vi "Convert 8SPC to 16SPC.vi"(0 "8xIQ in":T3=[{"I"=0.0, "Q"=0.0, "overflow"=FALSE}, {"I"=0.0, "Q"=0.0, "overflow"=FALSE}, {"I"=0.0, "Q"=0.0, "overflow"=FALSE}, {"I"=0.0, "Q"=0.0, "overflow"=FALSE}, {"I"=0.0, "Q"=0.0, "overflow"=FALSE}, {"I"=0.0, "Q"=0.0, "overflow"=FALSE}, {"I"=0.0, "Q"=0.0, "overflow"=FALSE}, {"I"=0.0, "Q"=0.0, "overflow"=FALSE}], 9 "input valid":bool=TRUE) -> (4 "16xIQ out":T1, 10 "output valid":bool=TRUE)   [LabVIEW 2015, in "DDC_7976R_v1.lvlib"]
uses:
  DDC_7976R_v1.lvlib
  Private/8xIQData.ctl
  <instrlib>/_niInstr/DSP/v1/Shared/Public/IQ Data.ctl
  Private/16xIQData.ctl
  <instrlib>/_niInstr/Basic Elements/v1/FPGA/niInstr Basic Elements v1 FPGA.lvlib
  <instrlib>/_niInstr/DSP/v1/Shared/niInstr DSP v1 Shared.lvlib
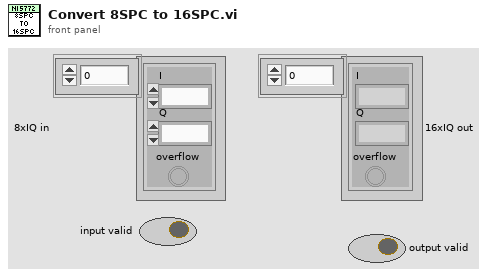
[diagram p1: front panel]
types:
  T1 = typedef "DDC_7976R_v1.lvlib/16xIQData.ctl" = T2[]
  T2 = typedef "niInstr DSP v1 Shared.lvlib/IQ Data.ctl" = cluster{"I":fxp<+/-,18,1>, "Q":fxp<+/-,18,1>, "overflow":bool}
  T3 = typedef "DDC_7976R_v1.lvlib/8xIQData.ctl" = T2[]
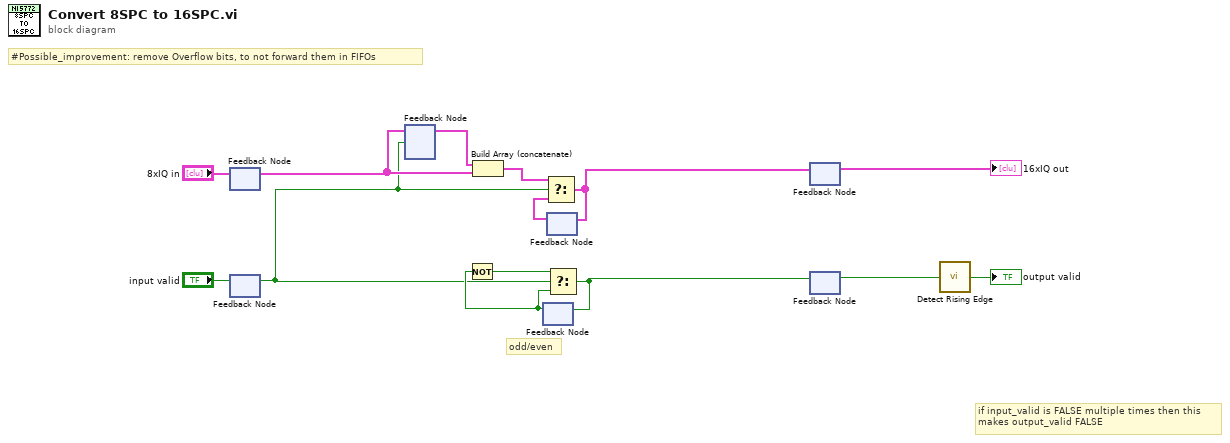
[diagram p0: block diagram]
diagram:
  # "odd/even"
  # "#Possible_improvement: remove Overflow bits, to not forward them in FIFOs"
  # "if input_valid is FALSE multiple times then this\nmakes output_valid FALSE"
  n1 = feedback #1() -> (w11:T3)  [unwired: 1 in]
  n2 = feedback-in #1("8xIQ in") -> ()
  n3 = feedback #2() -> (w1:bool)  [unwired: 1 in]
  n4 = feedback-in #2("input valid") -> ()
  n5 = feedback #3() -> (w8:T3)  [unwired: 1 in]
  n6 = feedback-in #3(w11, w1) -> ()
  n7 = Build Array (concatenate)(w8, w11) -> (w7:T2[])
  n8 = feedback #4() -> (w3:bool)  [unwired: 1 in]
  n9 = Not(x=w3) -> (.not. x?=w4:bool)
  n10 = feedback #5() -> (w6:T2[])  [unwired: 1 in]
  n11 = Select(t=w7, s=w1, f=w6) -> (s? t:f=w5:T2[])
  n12 = feedback-in #5(w5) -> ()
  n13 = Select(t=w4, s=w1, f=w3) -> (s? t:f=w2:bool)
  n14 = feedback-in #4(w2) -> ()
  n15 = feedback #6() -> (→"16xIQ out":T2[])  [unwired: 1 in]
  n16 = feedback-in #6(w5) -> ()
  n17 = feedback #7() -> (w14:bool)  [unwired: 1 in]
  n18 = feedback-in #7(w2) -> ()
  n19 = call <instrlib>:"Detect Rising Edge.vi"("signal"=w14) -> ("edge detected"=→"output valid":bool)  [unwired: 14 in]
